vi "create tls http server.vi"(8 "error in":errorcluster) -> (0 "error out":errorcluster, 3 "TLS HTTP server out":refnum<class "TLS HTTP server.lvclass">)   [LabVIEW 2016, in "TLS HTTP server.lvclass"]
uses:
  TLS HTTP server.lvclass
  TLS HTTP server.lvclass/TLS HTTP server.ctl
  lvlibtls/server/lvlibretls server listener.lvclass
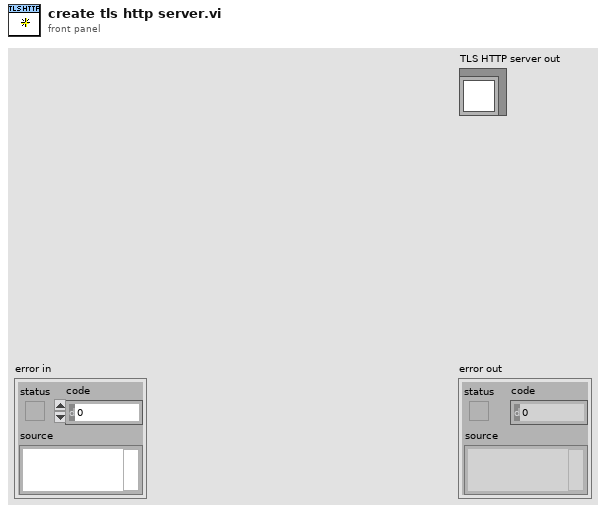
[diagram p1: front panel]
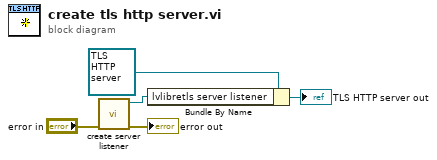
[diagram p0: block diagram]
diagram:
  n1 = call "create server listener.vi"("error in"="error in") -> ("error out"=→"error out":errorcluster, "lvlibretls server listener out"=w1:refnum<class "lvlibretls server listener.lvclass">)  [unwired: 9 in]
  n2 = Bundle By Name(cluster=refnum<class "TLS HTTP server.lvclass"> refnum ("TLS HTTP server in"), "lvlibretls server listener"=w1) -> (→"TLS HTTP server out":refnum<class "TLS HTTP server.lvclass">)
